vi "ErrorLog_Create.vi"(5 "Max File Size (1MB)":i32=1000000, 6 "ErrorLog FileName (\"Errors\")":string="Errors", 7 "Max Log Files (5)":i32=5, 8 "error in (no error)":errorcluster, 9 "Supress Consecutive Duplicates (T)":bool=TRUE, 10 "ErrorLog Folder (c:\\)":path=path "c:/", 11 "reference in":refnum<class "ErrorLog.lvclass">) -> (0 "error out":errorcluster, 3 "reference out":refnum<class "ErrorLog.lvclass">)   [LabVIEW 2014, in "ErrorLog.lvclass"]
uses:
  ErrorLog.lvclass
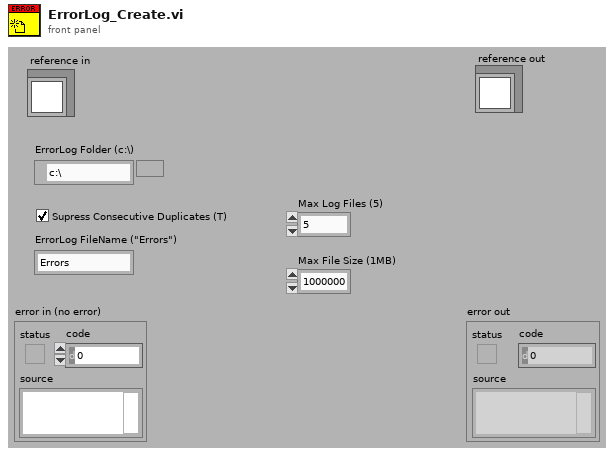
[diagram p1: front panel]
types:
  T1 = typedef "ErrorLog.lvclass/ObjectAttributes.ctl" = cluster{"ErrorFile":path, "Supress Consecutive Duplicates":bool, "Errors":string, "Quit":bool, "Errors since last call":string, "Last Recorded Error":string, "ErrorPath":path, "PossiblePaths":path[], "BaseFileName":string, "Max Log Files":i32, "ErrorFile Index":i32, "Max File Size":i64}
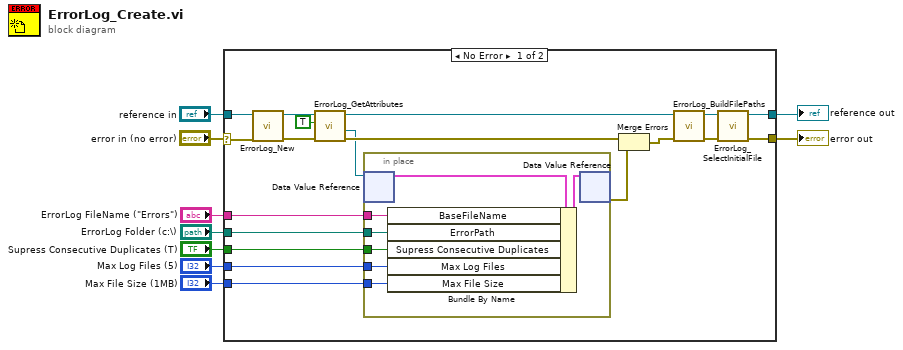
[diagram p0: block diagram]
diagram:
  n1 = case shown="No Error" "error in (no error)" {
    selector: "error in (no error)" -> [w24 w37]
    tunnel: [w12 w37] -> w9
    tunnel: "reference in" -> [w25 w36]
    tunnel: [w13 w36] -> w7
    tunnel: "ErrorLog Folder (c:\\)" -> [w22 _]
    tunnel: "Supress Consecutive Duplicates (T)" -> [w21 _]
    tunnel: "ErrorLog FileName (\"Errors\")" -> [w18 _]
    tunnel: "Max Log Files (5)" -> [w11 _]
    tunnel: "Max File Size (1MB)" -> [w10 _]
    frame No Error {
      n2 = call "ErrorLog_New.vi"("error in (no error)"=w24, "reference in"=w25) -> ("error out"=w27:errorcluster, "reference out"=w28:refnum<class "ErrorLog.lvclass">)  [unwired: 2 in, 6 out]
      n3 = call "ErrorLog_GetAttributes.vi"("error in (no error)"=w27, "OnlyGetDvrReference(False)"=TRUE, "reference in"=w28) -> ("error out"=w26:errorcluster, "DataRef"=w20:refnum<data-value>, "reference out"=w16:refnum<class "ErrorLog.lvclass">)  [unwired: 5 in, 1 out]
      n4 = in-place {
        in-place-border: w22 -> [w34]
        in-place-border: w21 -> [w33]
        in-place-border: w18 -> [w31]
        in-place-border: w11 -> [w30]
        in-place-border: w10 -> [w29]
        n5 = in-place-dvr #1(w20) -> (w35:T1)  [unwired: 1 out]
        n6 = Bundle By Name(cluster=w35, "BaseFileName"=w31, "ErrorPath"=w34, "Supress Consecutive Duplicates"=w33, "Max Log Files"=w30, "Max File Size"=w29) -> (w32:T1)
        n7 = in-place-dvr #1(w32) -> (w19:errorcluster)  [unwired: 1 out]
      }
      n8 = Merge Errors(w26, w19) -> (w17:errorcluster)
      n9 = call-dynamic "ErrorLog_BuildFilePaths.vi"("error in (no error)"=w17, "reference in"=w16) -> ("error out"=w15:errorcluster, "reference out"=w14:refnum<class "ErrorLog.lvclass">)  [unwired: 8 in]
      n10 = call-dynamic "ErrorLog_SelectInitialFile.vi"("error in (no error)"=w15, "reference in"=w14) -> ("error out"=w12:errorcluster, "reference out"=w13:refnum<class "ErrorLog.lvclass">)  [unwired: 8 in]
    }
    frame Error {
    }
  }
  "error out" <- w9
  "reference out" <- w7
